vi "Open Config File.vi"(6 "Create file if not found? (T)":bool=TRUE, 8 "error in (no error)":errorcluster, 11 "Path":path) -> (0 "error out":errorcluster, 2 "file created?":bool, 3 "file refnum":T1)   [LabVIEW 2019, in "TSC File IO.lvlib"]
doc: "This VI will open the configuration file and strip the ppl namespace if present.\n\nInputs:\n-Path [path] - a path to the file\n-error in\n\nOutputs:\n-file refnum [ref] - reference to the config file\n-error out\n\n<b>Code Developed By:</b>\nDaniel Coons\nTechnology Service Corporation\n1983 S Liberty Drive\nBloomington, IN 47403\nwww.tsc.com\\atcs"
uses:
  <vilib>/Utility/config.llb/Config Data RefNum.ctl
  TSC File IO.lvlib
  <vilib>/Utility/config.llb/NI_LVConfig.lvlib
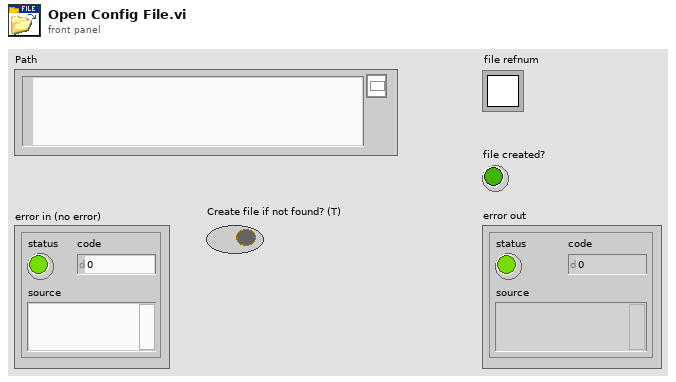
[diagram p1: front panel]
types:
  T1 = typedef "NI_LVConfig.lvlib/Config Data RefNum.ctl" = refnum<k1>
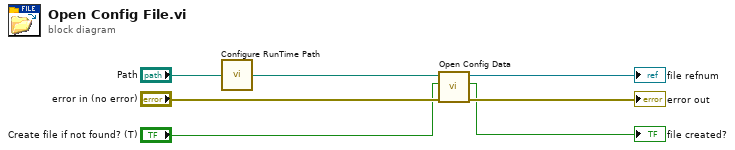
[diagram p0: block diagram]
diagram:
  n1 = call "Configure RunTime Path.vi"("Input Path"="Path") -> ("Updated Path"=w5:path)
  n2 = call <vilib>:"Open Config Data.vi"("error in (no error)"="error in (no error)", "create file if necessary (T)"="Create file if not found? (T)", "configuration file path"=w5) -> ("error out"=→"error out":errorcluster, "file created?"=→"file created?":bool, "refnum"=→"file refnum":T1)  [unwired: 6 in]
